vi "ErrorFGV.vi"(10 "error in (no error)":errorcluster) -> (2 "error out":errorcluster, 3 "SlaveLoopError":errorcluster)   [LabVIEW 2019, in "RT_Game.lvlib" / "Engine.lvclass"]
uses:
  Engine.lvclass
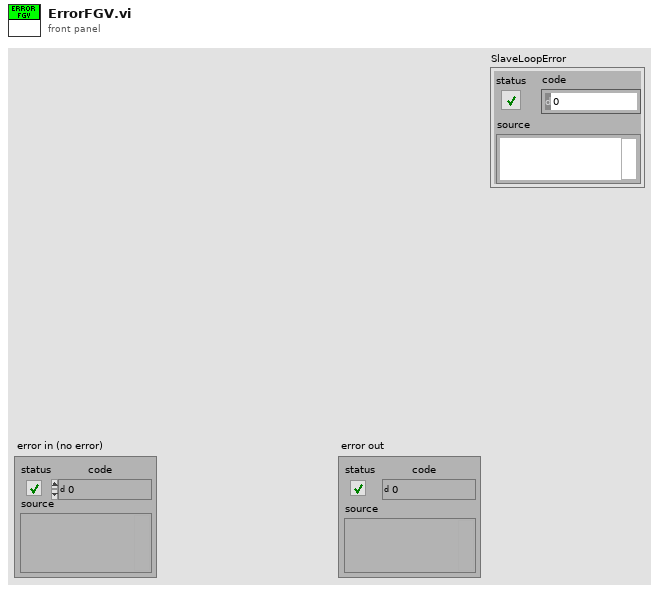
[diagram p1: front panel]
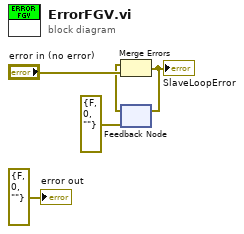
[diagram p0: block diagram]
diagram:
  n1 = feedback #1(errorcluster {"status"=FALSE, "code"=0, "source"=""} ("error IO")) -> (w1:errorcluster)
  n2 = Merge Errors(w1, "error in (no error)") -> (w5:errorcluster)
  "SlaveLoopError" <- w5
  n3 = feedback-in #1(w5) -> ()
  "error out" <- errorcluster {"status"=FALSE, "code"=0, "source"=""} ("error out")
